vi "Llamada a Api Extractor PDF.vi"() -> ()   [LabVIEW 2019]
uses:
  <vilib>/httpClient/POSTBuffer.vi
  <vilib>/httpClient/LabVIEWHTTPClient.lvlib
panel:
  out "body":string
  out "value":string[][](array[string])
  in  "PerfilId":string
  in  "Path_PDF":string
  out "headers":string
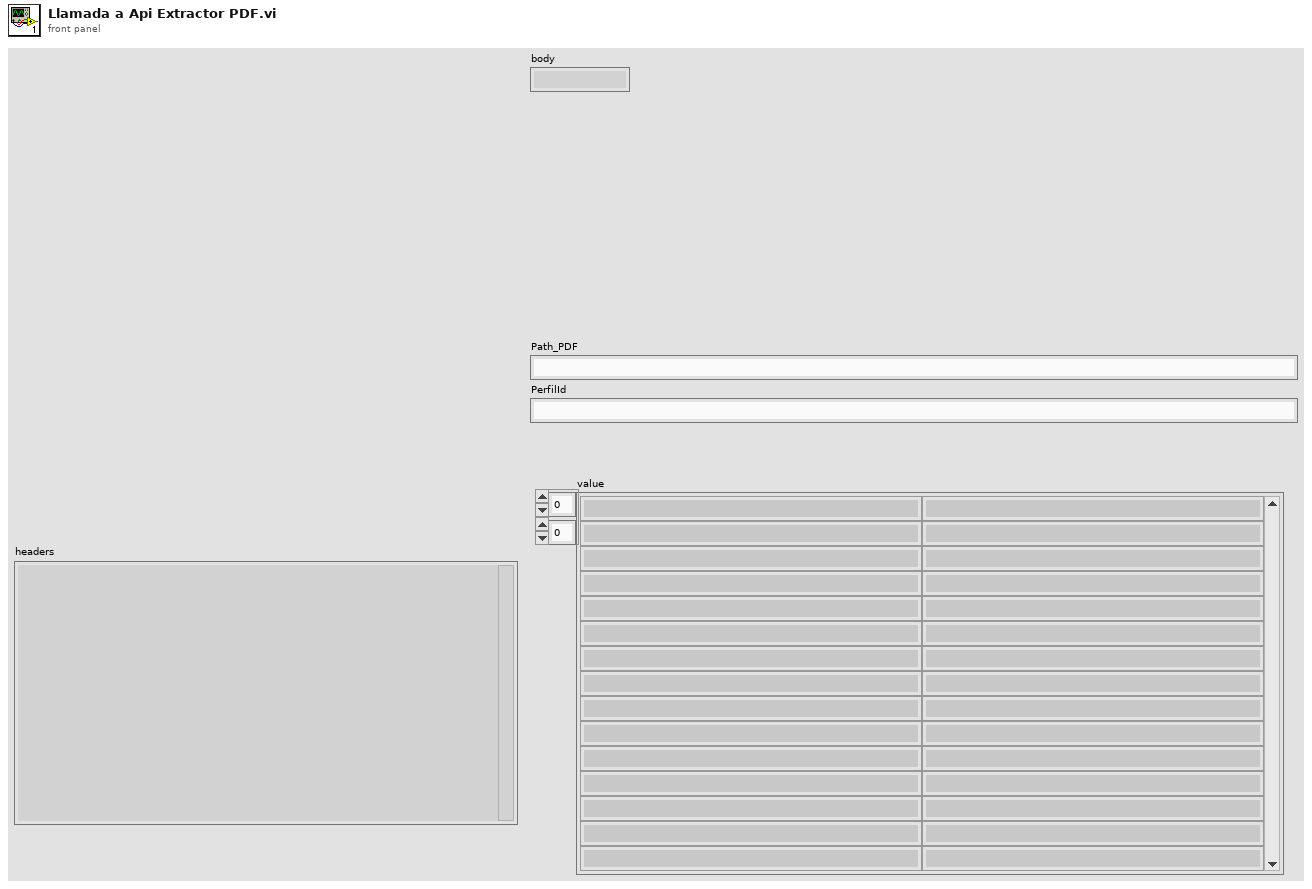
[diagram p1: front panel]
types:
  T1 = typedef "LabVIEWHTTPClient.lvlib/ClientHandle.ctl" = refnum<k1>
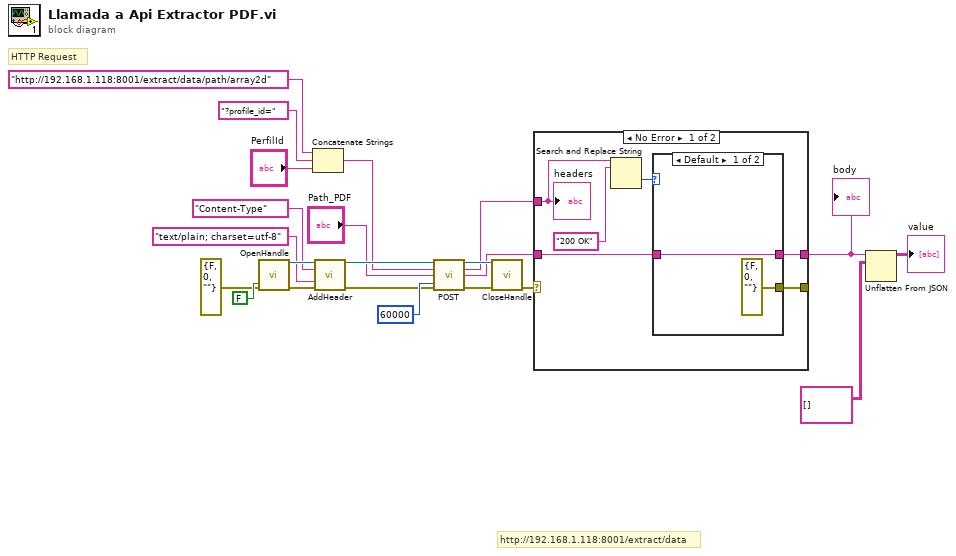
[diagram p0: block diagram]
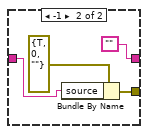
[diagram p2: hidden frame]
diagram:
  # "http://192.168.1.118:8001/extract/data"
  # "HTTP Request"
  n1 = call <vilib>:"OpenHandle.vi"("error in (no error)"=errorcluster {"status"=FALSE, "code"=0, "source"=""}, "verify server(true)"=FALSE) -> ("client handle out"=w15:T1, "error out"=w13:errorcluster)  [unwired: 12 in]
  n2 = Concatenate Strings("http://192.168.1.118:8001/extract/data/path/array2d", "?profile_id=" ("PerfilId"), "PerfilId") -> (w4:string)
  n3 = call <vilib>:"AddHeader.vi"("client handle"=w15, "header"="Content-Type", "value"="text/plain; charset=utf-8", "error in (no error)"=w13) -> ("client handle out"=w14:T1, "error out"=w12:errorcluster)  [unwired: 10 in]
  n4 = call-poly <vilib>:"POST.vi"("client handle"=w14, "url"=w4, "buffer"="Path_PDF", "error in (no error)"=w12, "timeout (10000)"=60000) -> ("client handle out"=w19:T1, "headers"=w18:string, "body"=w17:string, "error out"=w11:errorcluster)  [unwired: 7 in]
  n5 = call <vilib>:"CloseHandle.vi"("client handle"=w19, "error in (no error)"=w11) -> ("error out"=w20:errorcluster)  [unwired: 13 in]
  n6 = case shown="No Error" w20 {
    selector: w20 -> [_ w36]
    tunnel: w17 -> [w24 w35]
    tunnel: w18 -> [w28 _]
    tunnel: [w25 w36] -> _
    tunnel: [w23 w35] -> w3
    frame No Error {
      n7 = Search and Replace String(input string=w28, search string="200 OK") -> (offset past replacement=w26:i32)  [unwired: 6 in, 3 out]
      n8 = case shown="Default" w26 {
        tunnel: [errorcluster {"status"=FALSE, "code"=0, "source"=""} ("error IO") w33] -> w25
        tunnel: w24 -> [w30 w32]
        tunnel: [w30 ""] -> w23
        frame Default {
        }
        frame -1 {
          n9 = Bundle By Name(cluster=errorcluster {"status"=TRUE, "code"=0, "source"=""} ("error IO"), "source"=w32) -> (w33:errorcluster)
        }
      }
      "headers" <- w28
    }
    frame Error {
    }
  }
  "body" <- w3
  n10 = Unflatten From JSON(JSON string=w3, type and defaults=string[][] []) -> (value=→"value":string[][])  [unwired: 5 in, 1 out]
